vi "Build Send.vi"(8 "error in (no error)":errorcluster, 10 "Send VI":refnum<vi>, 11 "CS++Actor in":refnum<class "CS++Actor.lvclass">) -> (0 "error out":errorcluster, 3 "CS++Actor out":refnum<class "CS++Actor.lvclass">)   [LabVIEW 2014, in "CS++Actor.lvlib" / "CS++Actor.lvclass"]
doc: "Creates the send.vi of the new message."
uses:
  CS++Actor.lvclass
  CS++Actor.lvclass/CS++Actor.ctl
  <vilib>/Utility/traverseref.llb/TRef TravTarget.ctl
  <vilib>/LabVIEW Icon API/lv_icon/Classes/Icon/Icon.lvclass
  <vilib>/Utility/traverseref.llb/VI Scripting - Traverse.lvlib
  <vilib>/LabVIEW Icon API/LabVIEW Icon API.lvlib
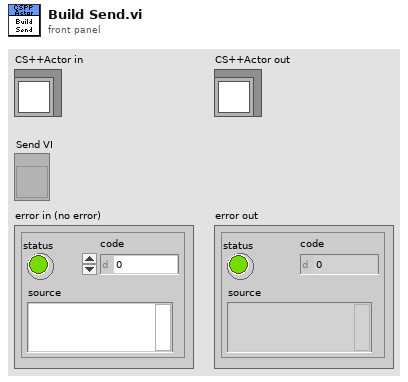
[diagram p1: front panel]
types:
  T1 = typedef "TRef TravTarget.ctl" = enum16{"FP", "BD", "Other"}
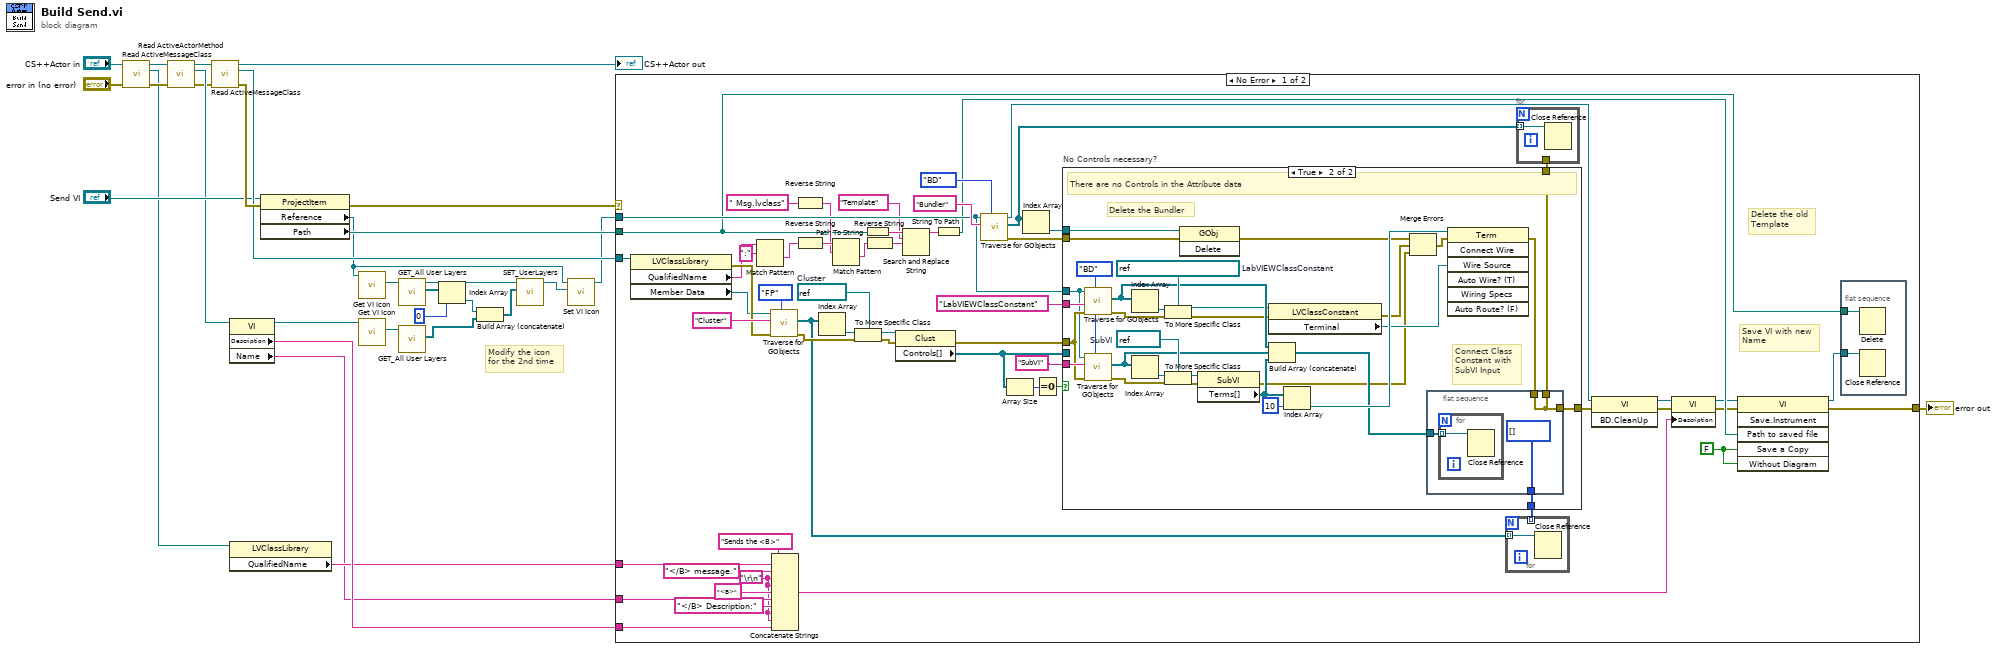
[diagram p0: block diagram]
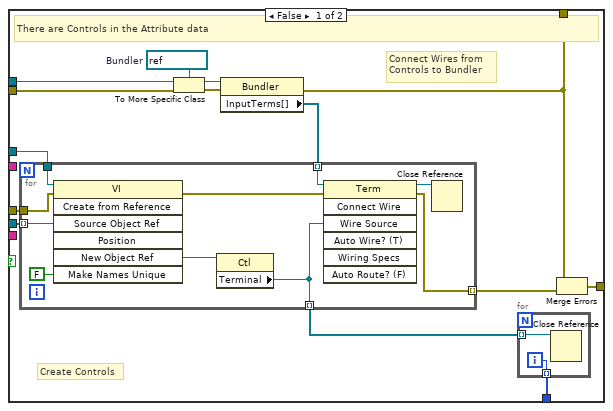
[diagram p2: hidden frame]
diagram:
  # "Modify the icon\nfor the 2nd time"
  n1 = call "Read ActiveMessageClass.vi"("error in (no error)"="error in (no error)", "CS++Actor in"="CS++Actor in") -> ("error out"=w4:errorcluster, "ActiveMessageClass"=w3:refnum<vi>, "CS++Actor out"=w6:refnum<class "CS++Actor.lvclass">)  [unwired: 7 in]
  n2 = call "Read ActiveActorMethod.vi"("error in (no error)"=w4, "CS++Actor in"=w6) -> ("error out"=w8:errorcluster, "ActiveActorMethod"=w12:refnum<vi>, "CS++Actor out"=w9:refnum<class "CS++Actor.lvclass">)  [unwired: 7 in]
  n3 = call "Read ActiveMessageClass.vi"("error in (no error)"=w8, "CS++Actor in"=w9) -> ("error out"=w26:errorcluster, "ActiveMessageClass"=w25:refnum<vi>, "CS++Actor out"=→"CS++Actor out":refnum<class "CS++Actor.lvclass">)  [unwired: 7 in]
  n4 = property class="VI"(reference=w12) -> (reference out=w11:refnum<vi>, "Description"=w10:string, "Name"=w1:string)  [unwired: 1 in, 1 out]
  n5 = property class="LVClassLibrary"(reference=w3) -> ("QualifiedName"=w2:string)  [unwired: 1 in, 2 out]
  n6 = property class="ProjectItem"(reference="Send VI", error in=w26) -> (error out=w29:errorcluster, "Reference"=w13:refnum<vi>, "Path"=w28:path)  [unwired: 1 out]
  n7 = call <vilib>:"Get VI Icon.vi"("VI Refnum in"=w13) -> ("Icon"=w22:refnum<class "Icon.lvclass">)  [unwired: 8 in, 2 out]
  n8 = call <vilib>:"Get VI Icon.vi"("VI Refnum in"=w11) -> ("Icon"=w21:refnum<class "Icon.lvclass">)  [unwired: 8 in, 2 out]
  n9 = call-dynamic "GET_All User Layers.vi"("Icon.lvclass in"=w22) -> ("User Layer"=w20:refnum<class "Layer.lvclass">[], "Icon.lvclass out"=w23:refnum<class "Icon.lvclass">)  [unwired: 8 in, 1 out]
  n10 = call-dynamic "GET_All User Layers.vi"("Icon.lvclass in"=w21) -> ("User Layer"=w17:refnum<class "Layer.lvclass">[])  [unwired: 8 in, 2 out]
  n11 = Index Array(array=w20, index=0) -> (element=w18:refnum<class "Layer.lvclass">)
  n12 = Build Array (concatenate)(w18, w17) -> (w16:refnum<class "Layer.lvclass">[])
  n13 = call-dynamic "SET_UserLayers.vi"("Layers"=w16, "Icon.lvclass in"=w23) -> ("Icon.lvclass out"=w15:refnum<class "Icon.lvclass">)  [unwired: 8 in, 1 out]
  n14 = call <vilib>:"Set VI Icon.vi"("Icon"=w15, "VI Refnum in"=w13) -> ("VI Refnum out"=w14:refnum<vi>)  [unwired: 8 in, 1 out]
  n15 = case shown="No Error" w29 {
    selector: w29 -> [_ w153]
    tunnel: [w52 w153] -> w30
    tunnel: w25 -> [w86 _]
    tunnel: w14 -> [w69 _]
    tunnel: w28 -> [w54 _]
    tunnel: w10 -> [w32 _]
    tunnel: w2 -> [w36 _]
    tunnel: w1 -> [w35 _]
    frame No Error {
      w31 = "\r\n"
      w68 = FALSE ("Save a Copy")
      w82 = refnum<vi> refnum  # Cluster
      # "Delete the old\nTemplate"
      # "Save VI with new\nName"
      n16 = property class="LVClassLibrary"(reference=w86) -> (error out=w80:errorcluster, "QualifiedName"=w62:string, "Member Data"=w63:refnum<vi>)  [unwired: 1 in, 1 out]
      n17 = Match Pattern(string=w62, regular expression=":") -> (after substring=w55:string)  [unwired: 1 in, 3 out]
      n18 = call <vilib>:"Traverse for GObjects.vi"("Traverse Target"=TRef_TravTarget."FP", "error in (no error)"=w80, "Class Name"="Cluster" ("name/order"), "VI Refnum"=w63) -> ("error out"=w81:errorcluster, "References"=w72:refnum<vi>[])  [unwired: 4 in, 2 out]
      n19 = Concatenate Strings("Sends the <B>", w36, "</B> message.", w31, w31, "<B>" ("string"), w35, "</B> Description:" ("string"), w31, w31, w32) -> (w39:string)
      n20 = Reverse String(1:" Msg.lvclass" ("search string")) -> (0:w57:string)
      n21 = Reverse String(1:w55) -> (0:w59:string)
      n22 = Index Array(array=w72) -> (element=w83:refnum<vi>)  [unwired: 1 in]
      n23 = Match Pattern(string=w59, regular expression=w57) -> (after substring=w58:string)  [unwired: 1 in, 3 out]
      n24 = To More Specific Class(target class=w82, reference=w83, error in=w81) -> (specific class reference=w79:refnum<vi>, error out=w78:errorcluster)
      n25 = Path To String(path=w54) -> (string=w67:string)
      n26 = Reverse String(1:w58) -> (0:w60:string)
      n27 = property class="Clust"(reference=w79, error in=w78) -> (error out=w77:errorcluster, "Controls[]"=w49:refnum<vi>[])  [unwired: 1 out]
      n28 = Search and Replace String(input string=w67, search string="Template", replace string=w60) -> (result string=w65:string)  [unwired: 5 in, 3 out]
      n29 = String To Path(string=w65) -> (path=w64:path)
      n30 = call <vilib>:"Traverse for GObjects.vi"("Traverse Target"=TRef_TravTarget."BD", "Class Name"="Bundler", "VI Refnum"=w69) -> ("error out"=w74:errorcluster, "References"=w71:refnum<vi>[], "dup VI Refnum"=w51:refnum<vi>)  [unwired: 5 in, 1 out]
      n31 = Array Size(array=w49) -> (size(s)=w48:i32)
      n32 = Index Array(array=w71) -> (element=w47:refnum<vi>)  [unwired: 1 in]
      n33 = Equal To 0?(x=w48) -> (x = 0?=w46:bool)
      n34 = case "No Controls necessary?" shown="True" w46 {
        tunnel: w77 -> [w100 w133]
        tunnel: w74 -> [w99 w143]
        tunnel: [w92 w140] -> w73
        tunnel: [w91 w141] -> w70
        tunnel: w69 -> [w90 w132]
        tunnel: [w89 w142] -> w50
        tunnel: w49 -> [w88 _]
        tunnel: w47 -> [w87 w144]
        tunnel: "LabVIEWClassConstant" ("Class Name") -> [_ w139]
        tunnel: "SubVI" ("Class Name") -> [_ w134]
        frame False {
          w98 = refnum<vi> refnum  # Bundler
          # "Connect Wires from\nControls to Bundler"
          # "Create Controls"
          # "There are Controls in the Attribute data"
          n35 = To More Specific Class(target class=w98, reference=w87, error in=w99) -> (specific class reference=w97:refnum<vi>, error out=w96:errorcluster)
          n36 = property class="Bundler"(reference=w97, error in=w96) -> (error out=w91:errorcluster, "InputTerms[]"=w95:refnum<vi>[])  [unwired: 1 out]
          n37 = for {
            tunnel: w88 -> [w112] mode=indexing
            tunnel: w90 -> [w110]
            tunnel: w100 -> [w109]
            tunnel: w95 -> [w107] mode=indexing
            tunnel: [w106] -> w94 mode=indexing
            tunnel: [w104] -> w93 mode=indexing
            n38 = invoke class="VI" method="Create from Reference"(reference=w110, error in=w109, "Source Object Ref"=w112, "Make Names Unique"=FALSE ("Make Names Unique (F)")) -> (error out=w108:errorcluster, "New Object Ref"=w105:refnum<vi>)  [unwired: 3 in, 5 out]
            n39 = property class="Ctl"(reference=w105) -> ("Terminal"=w104:refnum<vi>)  [unwired: 1 in, 2 out]
            n40 = invoke class="Term" method="Connect Wire"(reference=w107, error in=w108, "Wire Source"=w104) -> (reference out=w103:refnum<vi>, error out=w106:errorcluster)  [unwired: 4 in, 5 out]
            n41 = Close Reference(reference=w103) -> ()  [unwired: 1 in, 1 out]
          }
          n42 = for {
            tunnel: w93 -> [w102] mode=indexing
            tunnel: [w101] -> w92 mode=indexing
            i -> [w101]
            n43 = Close Reference(reference=w102) -> ()  [unwired: 1 in, 1 out]
          }
          n44 = Merge Errors(w91, w94) -> (w89:errorcluster)
        }
        frame True {
          w129 = refnum<vi> refnum  # SubVI
          w137 = refnum<vi> refnum  # LabVIEWClassConstant
          w135 = TRef_TravTarget."BD" ("Traverse Target")
          # "Connect Class\nConstant with\nSubVI Input"
          # "Delete the Bundler"
          # "There are no Controls in the Attribute data"
          n45 = call <vilib>:"Traverse for GObjects.vi"("Traverse Target"=w135, "error in (no error)"=w133, "Class Name"=w139, "VI Refnum"=w132) -> ("error out"=w136:errorcluster, "References"=w121:refnum<vi>[])  [unwired: 4 in, 2 out]
          n46 = call <vilib>:"Traverse for GObjects.vi"("Traverse Target"=w135, "error in (no error)"=w133, "Class Name"=w134, "VI Refnum"=w132) -> ("error out"=w130:errorcluster, "References"=w120:refnum<vi>[])  [unwired: 4 in, 2 out]
          n47 = Index Array(array=w121) -> (element=w138:refnum<vi>)  [unwired: 1 in]
          n48 = Index Array(array=w120) -> (element=w131:refnum<vi>)  [unwired: 1 in]
          n49 = To More Specific Class(target class=w137, reference=w138, error in=w136) -> (specific class reference=w117:refnum<vi>, error out=w115:errorcluster)
          n50 = To More Specific Class(target class=w129, reference=w131, error in=w130) -> (specific class reference=w128:refnum<vi>, error out=w127:errorcluster)
          n51 = invoke class="GObj" method="Delete"(reference=w144, error in=w143) -> (error out=w124:errorcluster)  [unwired: 1 in, 2 out]
          n52 = property class="SubVI"(reference=w128, error in=w127) -> (error out=w113:errorcluster, "Terms[]"=w119:refnum<vi>[])  [unwired: 1 out]
          n53 = property class="LVClassConstant"(reference=w117, error in=w115) -> (error out=w114:errorcluster, "Terminal"=w116:refnum<vi>)  [unwired: 1 out]
          n54 = Build Array (concatenate)(w121, w120, w119) -> (w118:refnum<vi>[])
          n55 = Index Array(array=w119, index=10) -> (element=w125:refnum<vi>)
          n56 = Merge Errors(w124, w114, w113) -> (w123:errorcluster)
          n57 = flat-sequence {
            tunnel: [w145] -> w142
            tunnel: [w145] -> w141
            tunnel: [i32[] []] -> w140
            tunnel: w122 -> [w145]
            tunnel: w118 -> [w146]
            frame #0 {
              n58 = for {
                tunnel: w146 -> [w148] mode=indexing
                n59 = Close Reference(reference=w148) -> ()  [unwired: 1 in, 1 out]
              }
            }
          }
          n60 = invoke class="Term" method="Connect Wire"(reference=w125, error in=w123, "Wire Source"=w116) -> (error out=w122:errorcluster)  [unwired: 4 in, 6 out]
        }
      }
      n61 = for {
        tunnel: w72 -> [w152] mode=indexing
        tunnel: w73 -> [_] mode=indexing
        n62 = Close Reference(reference=w152) -> ()  [unwired: 1 in, 1 out]
      }
      n63 = for {
        tunnel: w71 -> [w151] mode=indexing
        tunnel: w70 -> [_]
        n64 = Close Reference(reference=w151) -> ()  [unwired: 1 in, 1 out]
      }
      n65 = invoke class="VI" method="BD.CleanUp"(reference=w51, error in=w50) -> (reference out=w43:refnum<vi>, error out=w41:errorcluster)  [unwired: 1 in, 1 out]
      n66 = property class="VI"(reference=w43, error in=w41, "Description"=w39) -> (reference out=w42:refnum<vi>, error out=w40:errorcluster)
      n67 = invoke class="VI" method="Save.Instrument"(reference=w42, error in=w40, "Path to saved file"=w64, "Save a Copy"=w68, "Without Diagram"=w68) -> (reference out=w53:refnum<vi>, error out=w52:errorcluster)  [unwired: 1 in, 4 out]
      n68 = flat-sequence {
        tunnel: w53 -> [w150]
        tunnel: w54 -> [w149]
        frame #0 {
          n69 = Delete(path (use dialog)=w149) -> ()  [unwired: 4 in, 3 out]
          n70 = Close Reference(reference=w150) -> ()  [unwired: 1 in, 1 out]
        }
      }
    }
    frame Error {
    }
  }
  "error out" <- w30
